vi "Init.vi"(8 "error in (no error)":errorcluster, 10 "Channel":i16, 11 "TrialBasedExperiment in":refnum<class "MouseBar.lvclass">) -> (0 "error out":errorcluster, 3 "TrialBasedExperiment out":refnum<class "MouseBar.lvclass">)   [LabVIEW 2014, in "MouseBar.lvclass"]
uses:
  MouseBar.lvclass
  Trial Based Experiment Statechart/PassiveExperiment/PassiveExperiment.lvclass
  Matlab API/Matlab API.lvlib
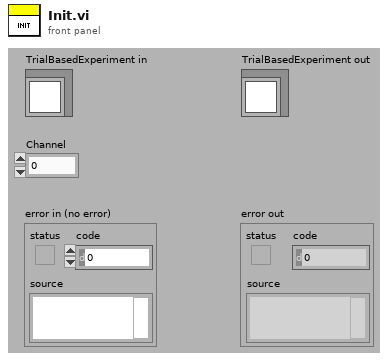
[diagram p1: front panel]
types:
  T1 = cluster{"Intertrial":dbl, "AcquireFixation":dbl, "HoldFixation":dbl, "DelayPeriod":dbl, "ResponsePeriod":dbl}
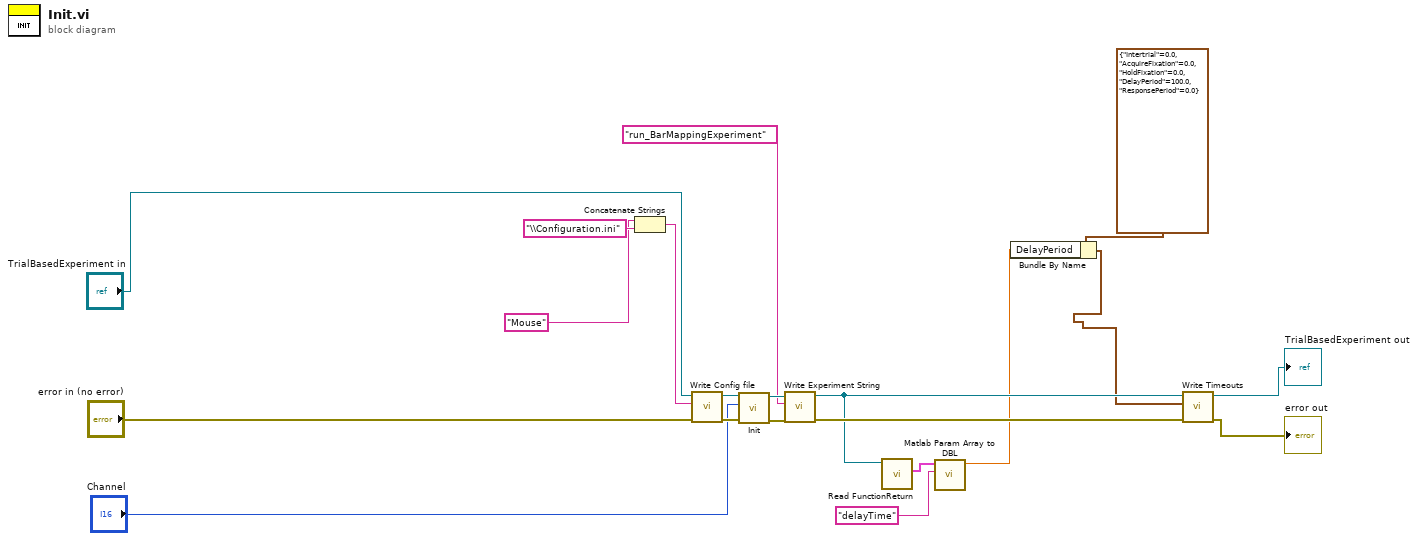
[diagram p0: block diagram]
diagram:
  n1 = Concatenate Strings("Mouse", "\\Configuration.ini") -> (w19:string)
  n2 = call-dynamic "Write Config file.vi"("error in (no error)"="error in (no error)", "Config file"=w19, "TrialBasedExperiment in"="TrialBasedExperiment in") -> ("error out"=w16:errorcluster, "TrialBasedExperiment out"=w18:refnum<class "MouseBar.lvclass">)  [unwired: 7 in]
  n3 = call-parent "Init.vi"("error in (no error)"=w16, "Channel"="Channel", "TrialBasedExperiment in"=w18) -> ("error out"=w15:errorcluster, "TrialBasedExperiment out"=w17:refnum<class "MouseBar.lvclass">)  [unwired: 7 in]
  n4 = call-dynamic "Write Experiment String.vi"("error in (no error)"=w15, "Experiment String"="run_BarMappingExperiment" ("string"), "TrialBasedExperiment in"=w17) -> ("error out"=w12:errorcluster, "TrialBasedExperiment out"=w7:refnum<class "MouseBar.lvclass">)  [unwired: 7 in]
  n5 = call-dynamic "Read FunctionReturn.vi"("MatlabExperiment in"=w7) -> ("FunctionReturn"=w6:cluster{"Name":string, "Data":variant}[])  [unwired: 8 in, 2 out]
  n6 = call "Matlab Param Array to DBL.vi"("Name"="delayTime", "Matlab Param Array"=w6) -> ("data"=w4:dbl)  [unwired: 8 in, 1 out]
  n7 = Bundle By Name(cluster=T1 {"Intertrial"=0.0, "AcquireFixation"=0.0, "HoldFixation"=0.0, "DelayPeriod"=100.0, "ResponsePeriod"=0.0} ("Timeouts"), "DelayPeriod"=w4) -> (w1:T1)
  n8 = call-dynamic "Write Timeouts.vi"("error in (no error)"=w12, "Timeouts"=w1, "TrialBasedExperiment in"=w7) -> ("error out"=→"error out":errorcluster, "TrialBasedExperiment out"=→"TrialBasedExperiment out":refnum<class "MouseBar.lvclass">)  [unwired: 7 in]
